vi "blurQuantifier.vi"() -> (0 "error out":errorcluster, 3 "Numeric":dbl)   [LabVIEW 2022 SP3]
panel:
  in  "error in":errorcluster
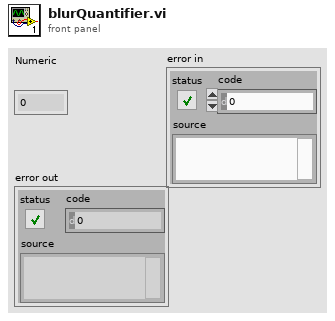
[diagram p1: front panel]
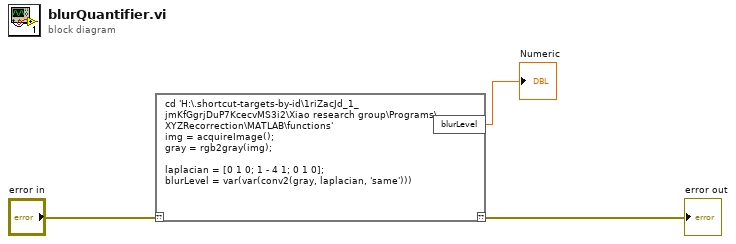
[diagram p0: block diagram]
diagram:
  n1 = script code="cd 'H:\\.shortcut-targets-by-id\\1riZacJd_1_jmKfGgrjDuP7KcecvMS3i2\\Xiao research group\\Programs\\XYZRecorrection\\MATLAB\\functions'\nimg = acquireImage();\ngray = rgb2gray(img);\n\nlaplacian = [0 1 0; 1 - 4 1; 0 1 0];\nblurLevel = var(var(conv2(gray, laplacian, 'same')))"("??"="error in") -> ("??"=→"error out":errorcluster, "blurLevel"=→"Numeric":dbl)
